vi "RD Analog Out Configure.vi"(8 "error in (no error)":errorcluster caption="错误输入（无错误）", 9 "output":bool, 10 "ch":i32, 11 "handle":u64) -> (0 "error out":errorcluster caption="错误输出", 2 "function return":i32, 3 "handle out":u64)   [LabVIEW 2018, in "InstrumentsPlayground.lvlib"]
doc: "CLIFFAPI int CliffAnalogOutConfigure(FT_HANDLE handle, int ch, bool output);\nch: 0 :ch1; 1 : ch2； 2：CH1&CH2"
uses:
  InstrumentsPlayground.lvlib
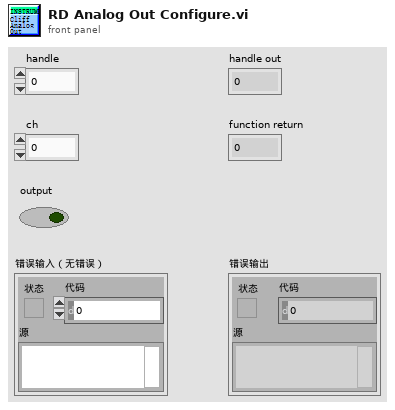
[diagram p1: front panel]
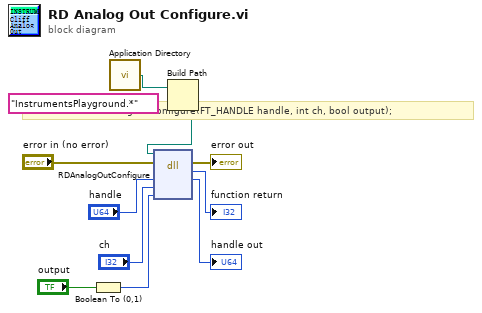
[diagram p0: block diagram]
diagram:
  # "CLIFFAPI int CliffAnalogOutConfigure(FT_HANDLE handle, int ch, bool output);"
  n1 = Boolean To (0,1)(Boolean="output") -> (0, 1=w6:i16)
  n2 = call <vilib>:"Application Directory.vi"() -> ("Application Directory"=w2:path)
  n3 = Build Path(base path=w2, name or relative path="InstrumentsPlayground.*" ("名称或相对路径")) -> (appended path=w1:path)
  n4 = dll-call lib="E:/work/YZCourse_Xtext/Cliff/API/LabVIEW lib/InstrumentsPlayground.*" fn="RDAnalogOutConfigure"(path in=w1, error in="error in (no error)", "handle"="handle", "ch"="ch", "output"=w6) -> (error out=→"error out":errorcluster, "返回类型"=→"function return":i32, "handle"=→"handle out":u64)  [unwired: 3 in, 1 out]
